vi "Example.vi"() -> ()   [LabVIEW 2012, in "AnalogDiscSDKLv.lvlib"]
uses:
  <instrlib>/AnalogDiscSDKLv/AnalogDiscSDKLv.lvlib
panel:
  out "Array":u8[](array[numeric])
  out "psts":u8
  out "initialized array":dbl[](array[numeric])
  out "Numeric":i32
  out "function return 7":i32
  out "size(s) 2":i32
  out "size(s)":i32
  out "rgdSamples out":dbl[](graph)
  out "hdwf":i32
  out "DeviceID":i32[](array[numeric])
  out "UserName":string
  out "SN":string
  out "DevName":string
  out "pnDevice":i32
  out "isBusy":i32[](array[numeric])
  out "DeviceVersion":i32[](array[numeric])
  out "function return 6":i32
  out "function return 5":i32
  out "function return 4":i32
  out "function return 3":i32
  out "function return 2":i32
  in  "indexCh":i32
  in  "Enable":i32=1
  in  "Filter":i32
  out "function return":i32
  in  "idxPin":i32
  in  "trigsrc":u8
  in  "voltOffset":dbl
  in  "voltsRange":dbl=5.0
  in  "nSize":i32=16384
  in  "hzFrquency":dbl=100000000.0 format="%#_6p"
  in  "AcqMode":i32
  in  "fStart":i32=1
  in  "fReconfigure":i32=1
  in  "fAutoConfig":i32=1
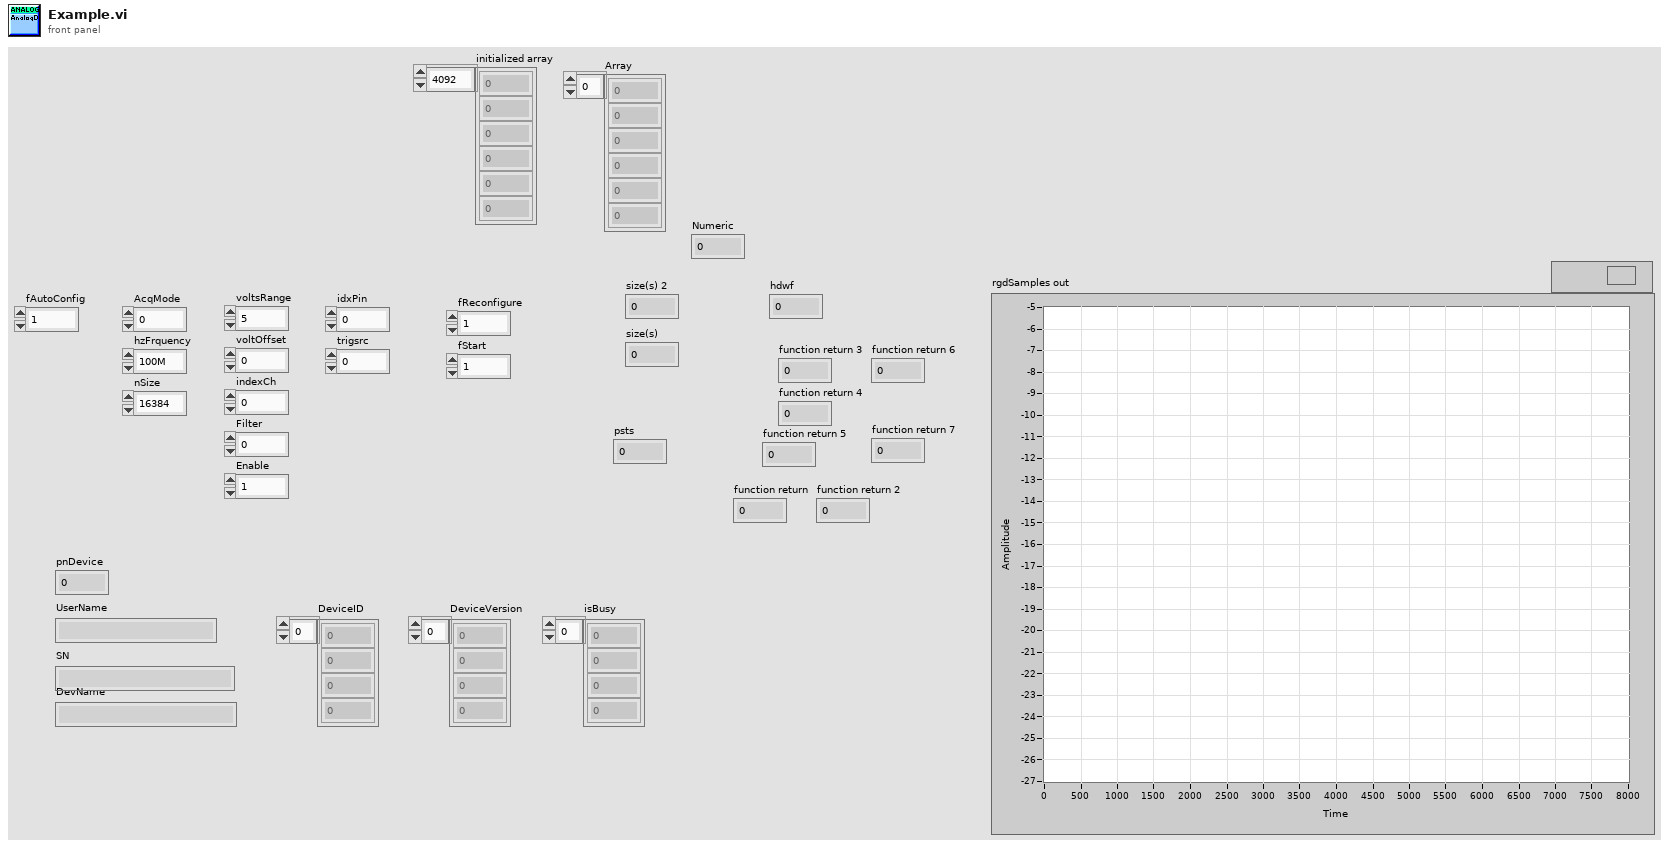
[diagram p1: front panel]
types:
  T1 = typedef "DWF_InstrumentStatus.ctl" = enum16{"stsRdy", "stsARM", "stsDone", "stsTrig", "stsCfg", "stsPrefill", "stsNotDone", "stsTrigDly", "stsError", "stsBusy", "stsStop"}
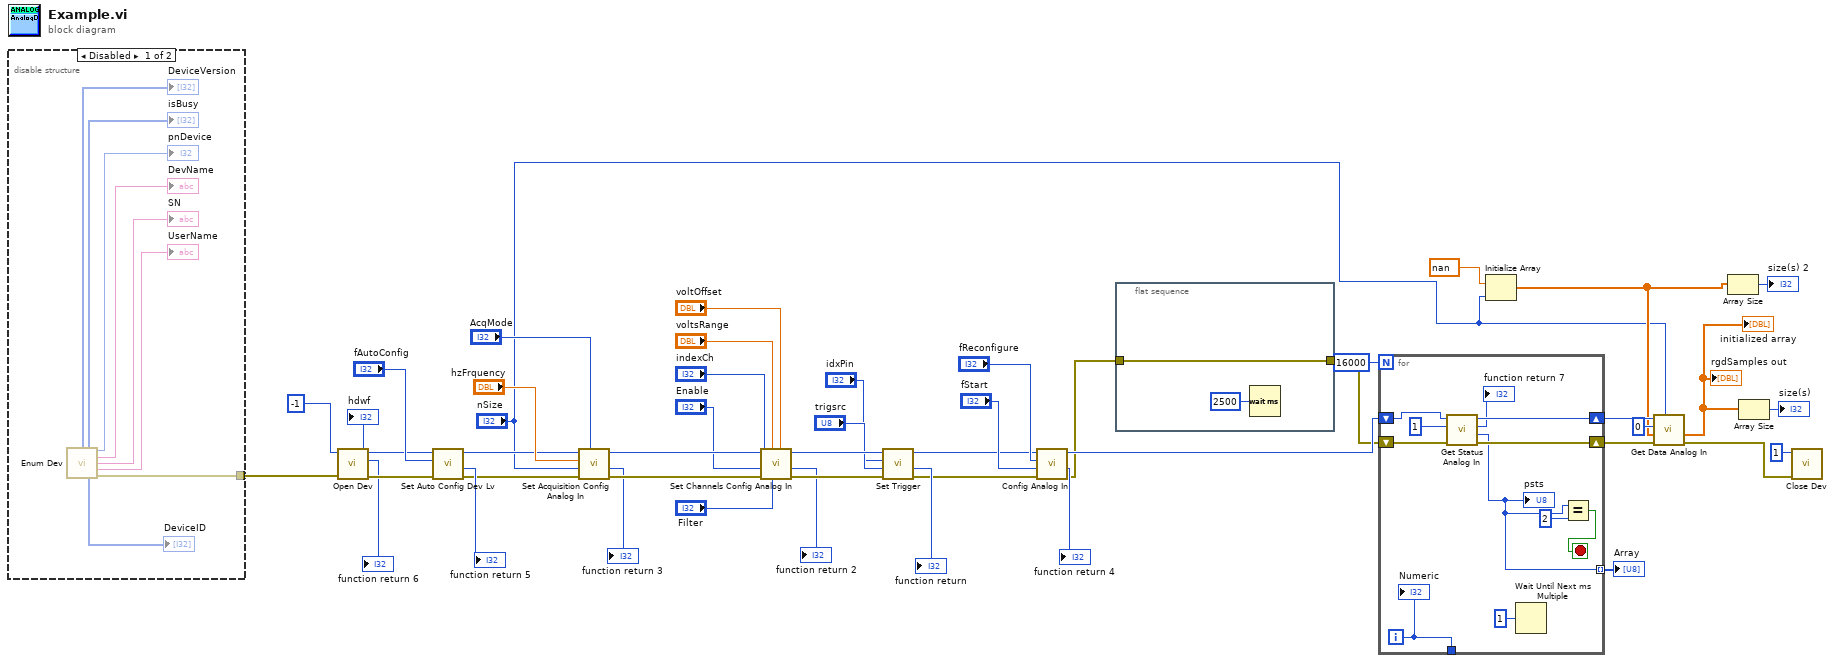
[diagram p0: block diagram]
diagram:
  n1 = disable-structure shown="Disabled" {
    disable-tunnel: [w54 _] -> w21
    frame Disabled {
      n2 = call <instrlib>:"Enum Dev.vi"() -> ("DeviceVersion"=→"DeviceVersion":i32[], "isBusy"=→"isBusy":i32[], "pnDevice"=→"pnDevice":i32, "DevName"=→"DevName":string, "SN"=→"SN":string, "UserName"=→"UserName":string, "DeviceID"=→"DeviceID":i32[], "error out"=w54:errorcluster)  [unwired: 7 in, 1 out]
    }
    frame Enabled {
    }
  }
  n3 = call <instrlib>:"Open Dev.vi"("error in (no error)"=w21, "idxDev"=-1) -> ("error out"=w43:errorcluster, "function return"=→"function return 6":i32, "hdwf"=w44:i32)  [unwired: 7 in]
  "hdwf" <- w44
  n4 = call <instrlib>:"Set Auto Config Dev Lv.vi"("error in (no error)"=w43, "fAutoConfig"="fAutoConfig", "hdwf"=w44) -> ("error out"=w20:errorcluster, "function return"=→"function return 5":i32, "hdwf out"=w19:i32)  [unwired: 6 in]
  n5 = call <instrlib>:"Set Acquisition Config Analog In.vi"("AcqMode"="AcqMode", "error in (no error)"=w20, "nSize"="nSize", "hzFrquency"="hzFrquency", "hdwf"=w19) -> ("error out"=w40:errorcluster, "function return"=→"function return 3":i32, "hdwf out"=w38:i32)  [unwired: 4 in]
  n6 = call <instrlib>:"Set Channels Config Analog In.vi"("voltOffset"="voltOffset", "Filter"="Filter", "voltsRange"="voltsRange", "error in (no error)"=w40, "Enable"="Enable", "indexCh"="indexCh", "hdwf"=w38) -> ("error out"=w39:errorcluster, "function return"=→"function return 2":i32, "hdwf out"=w33:i32)  [unwired: 2 in]
  n7 = call <instrlib>:"Set Trigger.vi"("error in (no error)"=w39, "trigsrc"="trigsrc", 10:"idxPin", "hdwf"=w33) -> ("error out"=w18:errorcluster, "function return"=→"function return":i32, "hdwf out"=w17:i32)  [unwired: 5 in]
  n8 = call <instrlib>:"Config Analog In.vi"("error in (no error)"=w18, "fStart"="fStart", "fReconfigure"="fReconfigure", "hdwf"=w17) -> ("error out"=w6:errorcluster, "function return"=→"function return 4":i32, "hdwf out"=w15:i32)  [unwired: 5 in]
  n9 = flat-sequence {
    tunnel: w6 -> [w55]
    tunnel: [w55] -> w5
    frame #0 {
      n10 = Wait (ms)(milliseconds to wait=u32 2500) -> ()  [unwired: 1 out]
    }
  }
  n11 = for {
    N: 16000 -> [_]
    shift-right: [w66] -> w14
    shift-left: w15 -> [w67]
    shift-right: [w64] -> w13
    shift-left: w5 -> [w63]
    tunnel: [w57] -> _
    tunnel: [w59] -> w2 mode=indexing
    i -> [w57]
    stop <- w60 stop-if-true
    n12 = call <instrlib>:"Get Status Analog In.vi"("error in (no error)"=w63, "fReadData"=1, "hdwf"=w67) -> ("error out"=w64:errorcluster, "psts"=w59:T1, "function return"=→"function return 7":i32, "hdwf out"=w66:i32)  [unwired: 4 in]
    "psts" <- w59
    n13 = Wait Until Next ms Multiple(millisecond multiple=u32 1) -> ()  [unwired: 1 out]
    n14 = Equal?(x=w59, y=u8 2) -> (x = y?=w60:bool)
    "Numeric" <- w57
  }
  "Array" <- w2
  n15 = Initialize Array(nan ("Numeric"), "nSize") -> (w7:dbl[])
  n16 = call <instrlib>:"Get Data Analog In.vi"("BufferSize"="nSize", "error in (no error)"=w13, "rgdSamples"=w7, "idxChannel"=0, "hdwf"=w14) -> ("error out"=w12:errorcluster, "rgdSamples out"=w4:dbl[])  [unwired: 4 in, 1 out]
  "rgdSamples out" <- w4
  "initialized array" <- w4
  n17 = Array Size(array=w7) -> (size(s)=→"size(s) 2":i32)
  n18 = Array Size(array=w4) -> (size(s)=→"size(s)":i32)
  n19 = call <instrlib>:"Close Dev.vi"("error in (no error)"=w12, "hdwf"=1) -> ()  [unwired: 8 in, 2 out]
